vi "test_Set and Get 9422.vi"(8 "error in (no error)":errorcluster, 11 "TestCase in":refnum<class "Scan Engine Scripting API Custom Device Unit Tests.lvclass">) -> (0 "error out":errorcluster, 3 "TestCase out":refnum<class "Scan Engine Scripting API Custom Device Unit Tests.lvclass">)   [LabVIEW 2017, in "Scan Engine Scripting API Custom Device Unit Tests.lvclass"]
uses:
  Scan Engine Scripting API Custom Device Unit Tests.lvclass
  Scan Engine Scripting API Custom Device Unit Tests.lvclass/Scan Engine Scripting API Custom Device Unit Tests.ctl
  Scripting/Modules/NI 9422/NI 9422.lvclass
  C:/dev/niveristand-scan-engine-ethercat-custom-device/Custom Device Source/Scripting/Modules/Module/Module.lvclass
  <vilib>/addons/_JKI Toolkits/VI Tester/TestCase.llb/TestCase.lvclass
  Scripting/Scan Engine Scripting.lvlib
  C:/Program Files (x86)/National Instruments/LabVIEW 2017/vi.lib/addons/_JKI Toolkits/VI Tester/TestCase.llb/TestCase.lvclass
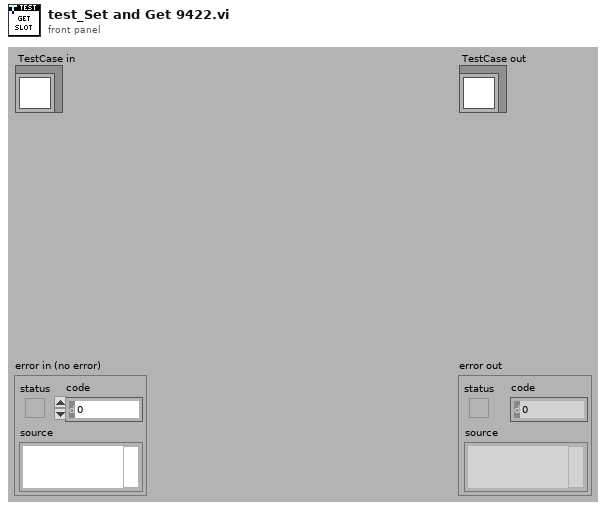
[diagram p1: front panel]
types:
  T1 = typedef "Custom Device API.lvlib/Custom Device Item Ref.ctl" = u64
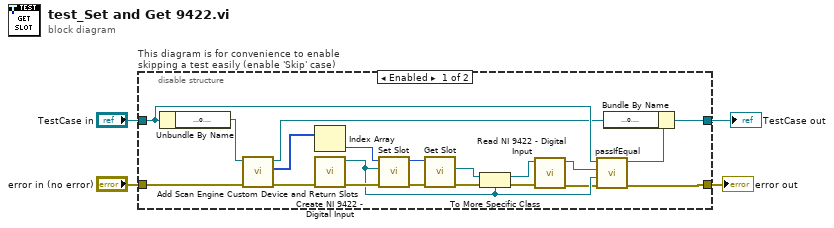
[diagram p0: block diagram]
diagram:
  n1 = disable-structure "This diagram is for convenience to enable skipping a test easily (enable 'Skip' case)" shown="Enabled" {
    disable-tunnel: "TestCase in" -> [w19 w28]
    disable-tunnel: [w23 w26] -> w1
    disable-tunnel: [w16 w27] -> w3
    disable-tunnel: "error in (no error)" -> [w7 w25]
    frame Enabled {
      n2 = Unbundle By Name(w19) -> ("target ref"=w9:refnum<k24>)
      n3 = call "Add Scan Engine Custom Device and Return Slots.vi"("error in"=w7, "target ref in"=w9) -> ("error out"=w6:errorcluster, "slot refs"=w8:T1[], "target ref out"=w5:refnum<k24>)  [unwired: 7 in]
      n4 = Index Array(array=w8) -> (element=w24:T1)  [unwired: 1 in]
      n5 = call "Create NI 9422 - Digital Input.vi"("error in"=w6) -> ("error out"=w18:errorcluster, "NI 9422 out"=w13:refnum<class "NI 9422.lvclass">)  [unwired: 9 in]
      n6 = call "Set Slot.vi"("error in"=w18, "module"=w13, "slot ref in"=w24) -> ("error out"=w22:errorcluster, "slot ref out"=w10:T1)  [unwired: 7 in]
      n7 = call "Get Slot.vi"("error in"=w22, "slot ref in"=w10) -> ("error out"=w21:errorcluster, "module"=w20:refnum<class "Module.lvclass">)  [unwired: 6 in, 2 out]
      n8 = To More Specific Class(target class=w13, reference=w20, error in=w21) -> (specific class reference=w15:refnum<class "NI 9422.lvclass">, error out=w17:errorcluster)
      n9 = call "Read NI 9422 - Digital Input.vi"("error in"=w17, "NI 9422 in"=w15) -> ("error out"=w12:errorcluster, "NI 9422 out"=w14:refnum<class "NI 9422.lvclass">)  [unwired: 7 in, 1 out]
      n10 = call-dynamic "passIfEqual.vi"("error in (no error)"=w12, "y"=w13, "x"=w14, "TestCase in"=w19) -> ("error out"=w16:errorcluster, "TestCase out"=w11:refnum<class "Scan Engine Scripting API Custom Device Unit Tests.lvclass">)  [unwired: 6 in]
      n11 = Bundle By Name(cluster=w11, "target ref"=w5) -> (w23:refnum<class "Scan Engine Scripting API Custom Device Unit Tests.lvclass">)
    }
    frame Disabled {
      # "skip test result while test is under development"
      n12 = call <vilib>:"skip.vi"("error in (no error)"=w25, "TestCase in"=w28) -> ("error out"=w27:errorcluster, "TestCase out"=w26:refnum<class "Scan Engine Scripting API Custom Device Unit Tests.lvclass">)  [unwired: 8 in]
    }
  }
  "error out" <- w3
  "TestCase out" <- w1
